vi "ReadTagValue.vi"(11 "Tag":T1) -> (0 "Number Read":dbl, 1 "Value Read":string)   [LabVIEW 2016, in "Systemlink Tag.xctl"]
uses:
  Systemlink Tag.xctl
  Systemlink Data.ctl
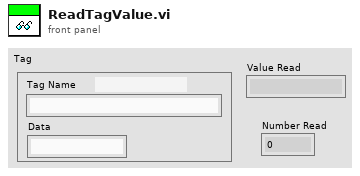
[diagram p1: front panel]
types:
  T1 = typedef "Systemlink Tag.xctl/Systemlink Data.ctl" = cluster{"Tag Name":string, "Type":string, "Data":string}
  T2 = typedef "SkylineCluster.ctl" = cluster{"Name":string, "BaseURL":string, "AppKey":string, "Headers":string[], "Timeout":i32}
  T3 = typedef "SystemLinkHTTPComm.ctl" = cluster{"url":string, "sent headers":string, "sent body":string, "headers":string, "body":string, "Sent":string, "Received":string}
  T4 = cluster{"current":cluster{"timestamp":string, "value":cluster{"type":string, "value":string}}}
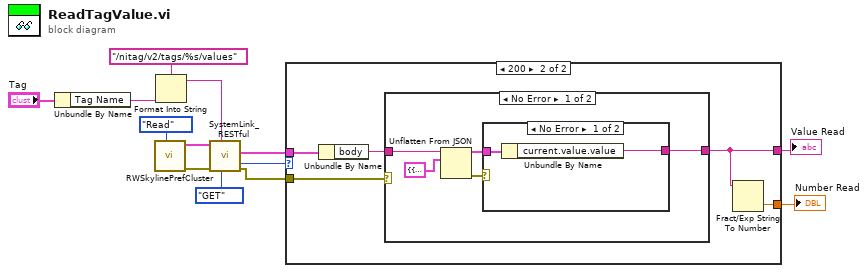
[diagram p0: block diagram]
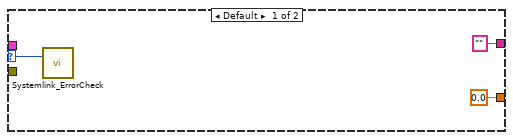
[diagram p2: hidden frame]
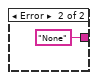
[diagram p3: hidden frame]
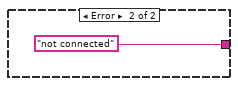
[diagram p4: hidden frame]
diagram:
  n1 = Unbundle By Name("Tag") -> ("Tag Name"=w7:string)
  n2 = call "RWSkylinePrefCluster.vi"("Task"=enum16{"Read", "Write"}."Read") -> ("error out"=w4:errorcluster, "Device Out"=w6:T2)  [unwired: 9 in]
  n3 = Format Into String(format string="/nitag/v2/tags/%s/values" ("url"), w7) -> (resulting string=w10:string)  [unwired: 2 in, 1 out]
  n4 = call "SystemLink_RESTful.vi"("Method"=enum16{"GET", "PUT", "POST", "MultiPOST"}."GET", "url"=w10, "error in"=w4, "Device In"=w6) -> ("error out"=w8:errorcluster, "HTTP Code"=w2:i32, "Comm"=w13:T3)  [unwired: 4 in, 1 out]
  n5 = case shown="200" w2 {
    selector: w2 -> [w16 _]
    tunnel: w13 -> [_ w21]
    tunnel: w8 -> [_ w19]
    tunnel: [0.0 w18] -> w3
    tunnel: ["" ("value") w17] -> w1
    frame Default {
      n6 = call "Systemlink_ErrorCheck.vi"("HTTP Code"=w16) -> ()  [unwired: 11 in]
    }
    frame 200 {
      n7 = Unbundle By Name(w21) -> ("body"=w20:string)
      n8 = case shown="No Error" w19 {
        tunnel: [w22 "not connected" ("value")] -> w17
        tunnel: w20 -> [w23 _]
        frame No Error {
          n9 = Unflatten From JSON(JSON string=w23, type and defaults=T4 {"current"={"timestamp"="", "value"={"type"="", "value"=""}}}) -> (value=w24:T4, error out=w25:errorcluster)  [unwired: 5 in]
          n10 = case shown="No Error" w25 {
            tunnel: w24 -> [w28 _]
            tunnel: [w27 "None" ("value")] -> w22
            frame No Error {
              n11 = Unbundle By Name(w28) -> ("current.value.value"=w27:string)
            }
            frame Error {
            }
          }
        }
        frame Error {
        }
      }
      n12 = Fract/Exp String To Number(string=w17) -> (number=w18:dbl)  [unwired: 3 in, 1 out]
    }
  }
  "Number Read" <- w3
  "Value Read" <- w1
